vi "Axis Not Mirorred.vi"(4 "Character Size":sgl=0.5, 5 "Half plane?":bool=TRUE, 6 "Axis label?":bool, 7 "Color":T1={"Red"=1.0, "Green"=0.0, "Blue"=0.0, "Alpha"=1.0}, 8 "error in (no error)":errorcluster, 9 "Radius":sgl=0.01, 10 "Length":sgl=2.0) -> (0 "error out":errorcluster, 3 "New Object Refnum":refnum<vi>)   [LabVIEW 2021]
uses:
  <vilib>/Utility/miscctls.llb/LVSceneTextAlignment.ctl
  <vilib>/picture/3D Picture Control/Object/Create Object (name).vi
  <vilib>/picture/3D Picture Control/Object/Create Object (drawable).vi
  <vilib>/picture/3D Picture Control/Object/Add Object (no reference).vi
  <vilib>/picture/3D Picture Control/NI_3D Picture Control.lvlib
panel:
  in  "Name":string="XYZ axis"
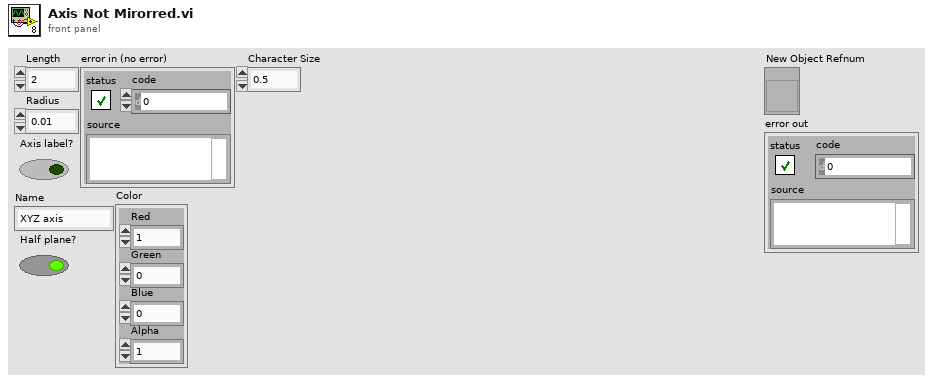
[diagram p1: front panel]
types:
  T1 = cluster{"Red":sgl, "Green":sgl, "Blue":sgl, "Alpha":sgl}
  T2 = typedef "LVSceneTextAlignment.ctl" = cluster{"Horizontal Alignment":enum8{"Left", "Right", "Center"}, "Vertical Alignment":enum8{"Top", "Bottom", "Center", "Base Line", "Bottom Base Line"}}
  T3 = cluster{"Alignment":T2, "Axis Alignment":enum8{"X-Y", "Y-Z", "X-Z", "Reversed X-Y", "Reversed Y-Z", "Reversed X-Z", "Screen"}, "Vertical?":bool, "Wrap Distance":sgl}
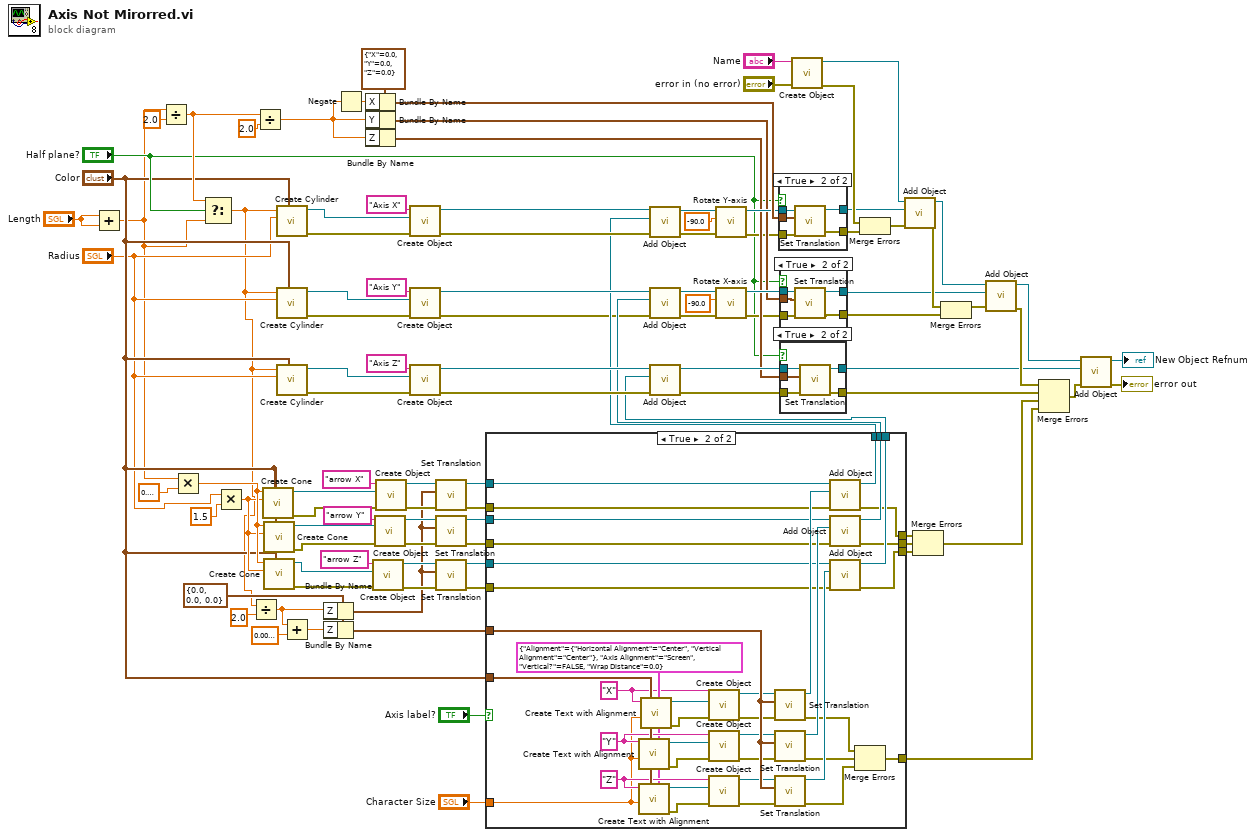
[diagram p0: block diagram]
diagram:
  w52 = cluster{"X":sgl, "Y":sgl, "Z":sgl} {"X"=0.0, "Y"=0.0, "Z"=0.0} ("Translation")
  w37 = cluster{"X":sgl, "Y":sgl, "Z":sgl} {"X"=0.0, "Y"=0.0, "Z"=0.0} ("Translation")
  n1 = Add(x="Length", y="Length") -> (x+y=w4:sgl)
  n2 = Divide(x=w4, y=sgl 2.0) -> (x/y=w73:sgl)
  n3 = Multiply(x=w4, y=sgl 0.1) -> (x*y=w15:sgl)
  n4 = Select(t=w73, s="Half plane?", f=w4) -> (s? t:f=w3:sgl)
  n5 = Multiply(x="Radius", y=sgl 1.5) -> (x*y=w14:sgl)
  n6 = Divide(x=w3, y=sgl 2.0 ("x")) -> (x/y=w16:sgl)
  n7 = Divide(x=w73, y=sgl 2.0) -> (x/y=w51:sgl)
  n8 = call <vilib>:"Create Cone.vi"("Color"="Color", "Radius"=w14, "Height"=w15) -> ("error out"=w17:errorcluster, "New Cone Refnum"=w59:refnum<vi>)  [unwired: 7 in]
  n9 = call <vilib>:"Create Cone.vi"("Color"="Color", "Radius"=w14, "Height"=w15) -> ("error out"=w9:errorcluster, "New Cone Refnum"=w11:refnum<vi>)  [unwired: 7 in]
  n10 = call <vilib>:"Create Cone.vi"("Color"="Color", "Radius"=w14, "Height"=w15) -> ("error out"=w10:errorcluster, "New Cone Refnum"=w12:refnum<vi>)  [unwired: 7 in]
  n11 = call <vilib>:"Create Cylinder.vi"("Color"="Color", "Radius"="Radius", "Height"=w3) -> ("error out"=w89:errorcluster, "New Cylinder Refnum"=w95:refnum<vi>)  [unwired: 7 in]
  n12 = call <vilib>:"Create Cylinder.vi"("Color"="Color", "Radius"="Radius", "Height"=w3) -> ("error out"=w88:errorcluster, "New Cylinder Refnum"=w97:refnum<vi>)  [unwired: 7 in]
  n13 = call <vilib>:"Create Cylinder.vi"("Color"="Color", "Radius"="Radius", "Height"=w3) -> ("error out"=w87:errorcluster, "New Cylinder Refnum"=w96:refnum<vi>)  [unwired: 7 in]
  n14 = Add(x=w16, y=sgl 0.01) -> (x+y=w28:sgl)
  n15 = Bundle By Name(cluster=w37, "Z"=w16) -> (w48:cluster{"X":sgl, "Y":sgl, "Z":sgl})
  n16 = Bundle By Name(cluster=w37, "Z"=w28) -> (w33:cluster{"X":sgl, "Y":sgl, "Z":sgl})
  n17 = Negate(x=w51) -> (-x=w1:sgl)
  n18 = Bundle By Name(cluster=w52, "X"=w1) -> (w75:cluster{"X":sgl, "Y":sgl, "Z":sgl})
  n19 = Bundle By Name(cluster=w52, "Y"=w51) -> (w53:cluster{"X":sgl, "Y":sgl, "Z":sgl})
  n20 = Bundle By Name(cluster=w52, "Z"=w51) -> (w50:cluster{"X":sgl, "Y":sgl, "Z":sgl})
  n21 = call-poly <vilib>:"Create Object.vi"("error in (no error)"=w10, "Geometry"=w12, "Name"="arrow Z") -> ("error out"=w60:errorcluster, "Scene:New Object"=w61:refnum<vi>)  [unwired: 7 in]
  n22 = call-poly <vilib>:"Create Object.vi"("error in (no error)"=w9, "Geometry"=w11, "Name"="arrow Y") -> ("error out"=w65:errorcluster, "Scene:New Object"=w64:refnum<vi>)  [unwired: 7 in]
  n23 = call-poly <vilib>:"Create Object.vi"("error in (no error)"=w17, "Geometry"=w59, "Name"="arrow X") -> ("error out"=w78:errorcluster, "Scene:New Object"=w79:refnum<vi>)  [unwired: 7 in]
  n24 = call-poly <vilib>:"Create Object.vi"("error in (no error)"=w89, "Geometry"=w95, "Name"="Axis X") -> ("error out"=w43:errorcluster, "Scene:New Object"=w68:refnum<vi>)  [unwired: 7 in]
  n25 = call-poly <vilib>:"Create Object.vi"("error in (no error)"=w88, "Geometry"=w97, "Name"="Axis Y") -> ("error out"=w20:errorcluster, "Scene:New Object"=w63:refnum<vi>)  [unwired: 7 in]
  n26 = call-poly <vilib>:"Create Object.vi"("error in (no error)"=w87, "Geometry"=w96, "Name"="Axis Z") -> ("error out"=w47:errorcluster, "Scene:New Object"=w58:refnum<vi>)  [unwired: 7 in]
  n27 = call <vilib>:"Set Translation.vi"("error in (no error)"=w78, "Translation"=w48, "Scene Object"=w79) -> ("error out"=w27:errorcluster, "Translated Object"=w39:refnum<vi>)  [unwired: 7 in]
  n28 = call <vilib>:"Set Translation.vi"("error in (no error)"=w65, "Translation"=w48, "Scene Object"=w64) -> ("error out"=w26:errorcluster, "Translated Object"=w36:refnum<vi>)  [unwired: 7 in]
  n29 = call <vilib>:"Set Translation.vi"("error in (no error)"=w60, "Translation"=w48, "Scene Object"=w61) -> ("error out"=w29:errorcluster, "Translated Object"=w34:refnum<vi>)  [unwired: 7 in]
  n30 = case shown="True" "Axis label?" {
    tunnel: w39 -> [w109 w146]
    tunnel: [w109 w145] -> w38
    tunnel: w36 -> [w108 w144]
    tunnel: [w108 w142] -> w35
    tunnel: w34 -> [w104 w141]
    tunnel: w33 -> [_ w140]
    tunnel: [w104 w138] -> w32
    tunnel: w29 -> [w106 w137]
    tunnel: w27 -> [w107 w136]
    tunnel: w26 -> [w105 w135]
    tunnel: [w107 w134] -> w25
    tunnel: [w105 w133] -> w24
    tunnel: [w106 w132] -> w23
    tunnel: [_ w131] -> w21
    tunnel: "Color" -> [_ w130]
    tunnel: "Character Size" -> [_ w110]
    frame False {
    }
    frame True {
      w122 = "Z" ("text")
      w127 = "Y" ("text")
      w117 = T3 {"Alignment"={"Horizontal Alignment"=enum."Center", "Vertical Alignment"=enum."Center"}, "Axis Alignment"=enum."Screen", "Vertical?"=FALSE, "Wrap Distance"=0.0} ("Font options")
      w115 = "X" ("text")
      n31 = call <vilib>:"Create Text with Alignment.vi"("Font Options"=w117, "Color"=w130, "Character Size"=w110, "Text"=w127) -> ("error out"=w119:errorcluster, "New Text Refnum"=w126:refnum<vi>)  [unwired: 6 in]
      n32 = call <vilib>:"Create Text with Alignment.vi"("Font Options"=w117, "Color"=w130, "Character Size"=w110, "Text"=w122) -> ("error out"=w121:errorcluster, "New Text Refnum"=w123:refnum<vi>)  [unwired: 6 in]
      n33 = call <vilib>:"Create Text with Alignment.vi"("Font Options"=w117, "Color"=w130, "Character Size"=w110, "Text"=w115) -> ("error out"=w114:errorcluster, "New Text Refnum"=w129:refnum<vi>)  [unwired: 6 in]
      n34 = call-poly <vilib>:"Create Object.vi"("error in (no error)"=w114, "Geometry"=w129, "Name"=w115) -> ("error out"=w116:errorcluster, "Scene:New Object"=w128:refnum<vi>)  [unwired: 7 in]
      n35 = call-poly <vilib>:"Create Object.vi"("error in (no error)"=w119, "Geometry"=w126, "Name"=w127) -> ("error out"=w118:errorcluster, "Scene:New Object"=w125:refnum<vi>)  [unwired: 7 in]
      n36 = call-poly <vilib>:"Create Object.vi"("error in (no error)"=w121, "Geometry"=w123, "Name"=w122) -> ("error out"=w120:errorcluster, "Scene:New Object"=w124:refnum<vi>)  [unwired: 7 in]
      n37 = call <vilib>:"Set Translation.vi"("error in (no error)"=w116, "Translation"=w140, "Scene Object"=w128) -> ("error out"=w111:errorcluster, "Translated Object"=w147:refnum<vi>)  [unwired: 7 in]
      n38 = call <vilib>:"Set Translation.vi"("error in (no error)"=w118, "Translation"=w140, "Scene Object"=w125) -> ("error out"=w112:errorcluster, "Translated Object"=w143:refnum<vi>)  [unwired: 7 in]
      n39 = call <vilib>:"Set Translation.vi"("error in (no error)"=w120, "Translation"=w140, "Scene Object"=w124) -> ("error out"=w113:errorcluster, "Translated Object"=w139:refnum<vi>)  [unwired: 7 in]
      n40 = call-poly <vilib>:"Add Object.vi"("error in (no error)"=w136, "New Object In"=w147, "Scene Object In"=w146) -> ("error out"=w134:errorcluster, "Scene Object Out"=w145:refnum<vi>)  [unwired: 7 in]
      n41 = call-poly <vilib>:"Add Object.vi"("error in (no error)"=w135, "New Object In"=w143, "Scene Object In"=w144) -> ("error out"=w133:errorcluster, "Scene Object Out"=w142:refnum<vi>)  [unwired: 7 in]
      n42 = call-poly <vilib>:"Add Object.vi"("error in (no error)"=w137, "New Object In"=w139, "Scene Object In"=w141) -> ("error out"=w132:errorcluster, "Scene Object Out"=w138:refnum<vi>)  [unwired: 7 in]
      n43 = Merge Errors(w111, w112, w113) -> (w131:errorcluster)
    }
  }
  n44 = call-poly <vilib>:"Add Object.vi"("error in (no error)"=w43, "New Object In"=w38, "Scene Object In"=w68) -> ("error out"=w42:errorcluster, "Scene Object Out"=w67:refnum<vi>)  [unwired: 7 in]
  n45 = call-poly <vilib>:"Add Object.vi"("error in (no error)"=w20, "New Object In"=w35, "Scene Object In"=w63) -> ("error out"=w19:errorcluster, "Scene Object Out"=w62:refnum<vi>)  [unwired: 7 in]
  n46 = call-poly <vilib>:"Add Object.vi"("error in (no error)"=w47, "New Object In"=w32, "Scene Object In"=w58) -> ("error out"=w46:errorcluster, "Scene Object Out"=w55:refnum<vi>)  [unwired: 7 in]
  n47 = call <vilib>:"Rotate Y-axis.vi"("error in (no error)"=w42, "angle"=-90.0, "Scene Object In"=w67) -> ("error out"=w41:errorcluster, "Scene Object Out"=w72:refnum<vi>)  [unwired: 7 in]
  n48 = call <vilib>:"Rotate X-axis.vi"("error in (no error)"=w19, "angle"=-90.0, "Scene Object In"=w62) -> ("error out"=w44:errorcluster, "Scene Object Out"=w57:refnum<vi>)  [unwired: 7 in]
  n49 = case shown="True" "Half plane?" {
    tunnel: w72 -> [w149 w154]
    tunnel: w75 -> [_ w153]
    tunnel: [w149 w152] -> w71
    tunnel: [w148 w151] -> w70
    tunnel: w41 -> [w148 w150]
    frame False {
    }
    frame True {
      n50 = call <vilib>:"Set Translation.vi"("error in (no error)"=w150, "Translation"=w153, "Scene Object"=w154) -> ("error out"=w151:errorcluster, "Translated Object"=w152:refnum<vi>)  [unwired: 7 in]
    }
  }
  n51 = case shown="True" "Half plane?" {
    tunnel: w57 -> [w156 w161]
    tunnel: [w156 w160] -> w56
    tunnel: [w155 w159] -> w49
    tunnel: w53 -> [_ w158]
    tunnel: w44 -> [w155 w157]
    frame False {
    }
    frame True {
      n52 = call <vilib>:"Set Translation.vi"("error in (no error)"=w157, "Translation"=w158, "Scene Object"=w161) -> ("error out"=w159:errorcluster, "Translated Object"=w160:refnum<vi>)  [unwired: 7 in]
    }
  }
  n53 = case shown="True" "Half plane?" {
    tunnel: w55 -> [w163 w168]
    tunnel: [w163 w167] -> w54
    tunnel: [w162 w166] -> w45
    tunnel: w50 -> [_ w165]
    tunnel: w46 -> [w162 w164]
    frame False {
    }
    frame True {
      n54 = call <vilib>:"Set Translation.vi"("error in (no error)"=w164, "Translation"=w165, "Scene Object"=w168) -> ("error out"=w166:errorcluster, "Translated Object"=w167:refnum<vi>)  [unwired: 7 in]
    }
  }
  n55 = call-poly <vilib>:"Create Object.vi"("error in (no error)"="error in (no error)", "Name"="Name") -> ("error out"=w86:errorcluster, "Scene:New Object"=w102:refnum<vi>)  [unwired: 8 in]
  n56 = Merge Errors(w86, w70) -> (w85:errorcluster)
  n57 = call-poly <vilib>:"Add Object.vi"("error in (no error)"=w85, "New Object In"=w71, "Scene Object In"=w102) -> ("error out"=w84:errorcluster, "Scene Object Out"=w101:refnum<vi>)  [unwired: 7 in]
  n58 = Merge Errors(w25, w24, w23) -> (w22:errorcluster)
  n59 = Merge Errors(w84, w49) -> (w83:errorcluster)
  n60 = call-poly <vilib>:"Add Object.vi"("error in (no error)"=w83, "New Object In"=w56, "Scene Object In"=w101) -> ("error out"=w82:errorcluster, "Scene Object Out"=w100:refnum<vi>)  [unwired: 7 in]
  n61 = Merge Errors(w82, w45, w22, w21) -> (w81:errorcluster)
  n62 = call-poly <vilib>:"Add Object.vi"("error in (no error)"=w81, "New Object In"=w54, "Scene Object In"=w100) -> ("error out"=→"error out":errorcluster, "Scene Object Out"=→"New Object Refnum":refnum<vi>)  [unwired: 7 in]
